vi "DSF.Engine.Framework.Number of Transceiver Threads.vi"(8 "error in (no error)":errorcluster, 10 "transceiver count":i32, 11 "Framework in":refnum<class "DSF.Engine.Framework.lvclass">) -> (0 "error out":errorcluster, 3 "Framework out":refnum<class "DSF.Engine.Framework.lvclass">)   [LabVIEW 2017, in "DSF.Engine.lvlib" / "DSF.Engine.Framework.lvclass"]
uses:
  DSF.Engine.Framework.lvclass
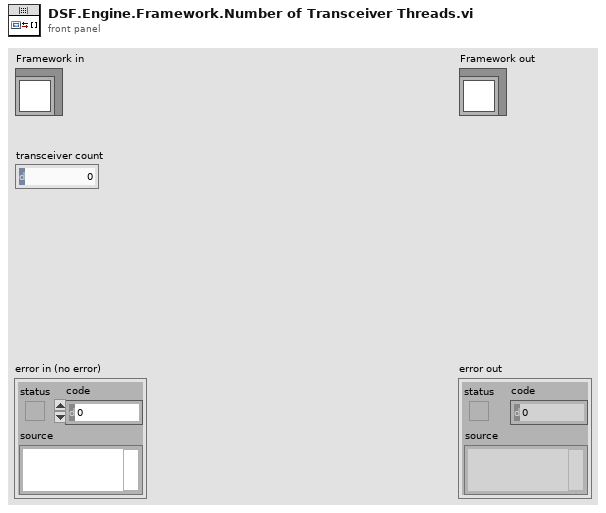
[diagram p1: front panel]
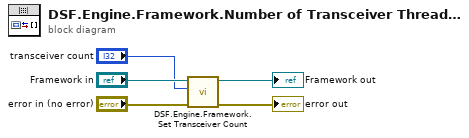
[diagram p0: block diagram]
diagram:
  n1 = call "DSF.Engine.Framework.Set Transceiver Count.vi"("transceiver count"="transceiver count", "Framework in"="Framework in") -> ("Framework out"=→"Framework out":refnum<class "DSF.Engine.Framework.lvclass">)  [unwired: 9 in]
  "error out" <- "error in (no error)"
